vi "ScanDelayGetTriggerOut.vi"(8 "error in (no error)":errorcluster, 9 "wait":u32=10, 11 "VISA resource name in":refnum<visa-resource-name>) -> (0 "error out":errorcluster, 2 "value":i32, 3 "VISA resource name out":refnum<visa-resource-name>)   [LabVIEW 2018]
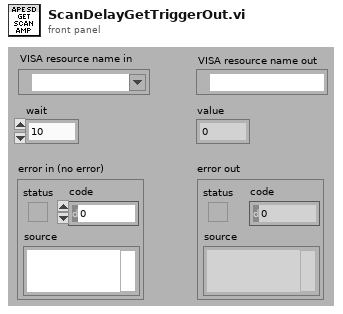
[diagram p1: front panel]
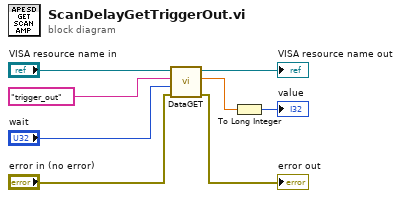
[diagram p0: block diagram]
diagram:
  n1 = call "DataGET.vi"("error in"="error in (no error)", "wait"="wait", "parameter"="trigger_out", "VISA resource name"="VISA resource name in") -> ("error out"=→"error out":errorcluster, "value"=w3:dbl, "VISA resource name out"=→"VISA resource name out":refnum<visa-resource-name>)  [unwired: 4 in]
  n2 = To Long Integer(number=w3) -> (32bit integer=→"value":i32)
